vi "labo01.04.radoslaw.wolnik.12.vi"() -> ()   [LabVIEW 2012]
panel:
  out "wartosc":string
  in  "Ciœnieniomierz":dbl(knob) scale=0.0..3500.0
  in  "Termometr":dbl(slide) scale=-20.0..100.0
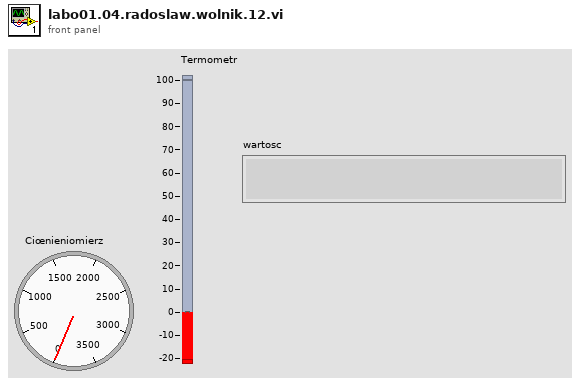
[diagram p1: front panel]
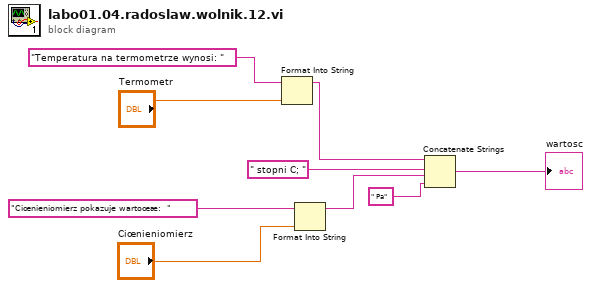
[diagram p0: block diagram]
diagram:
  n1 = Format Into String(initial string="Temperatura na termometrze wynosi: ", "Termometr") -> (resulting string=w7:string)  [unwired: 2 in, 1 out]
  n2 = Format Into String(initial string="Ciœnieniomierz pokazuje wartoœæ:  ", "Ciœnieniomierz") -> (resulting string=w3:string)  [unwired: 2 in, 1 out]
  n3 = Concatenate Strings(w7, " stopni C; ", w3, " Pa") -> (→"wartosc":string)
